vi "parse -- split by line.vi"() -> ()   [LabVIEW 2010]
panel:
  in  "regexp":string="(\\s*[\\d\\.\\+\\-]+)+\\s*\\r?"
  in  "string array":string[](array[string])
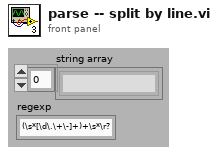
[diagram p1: front panel]
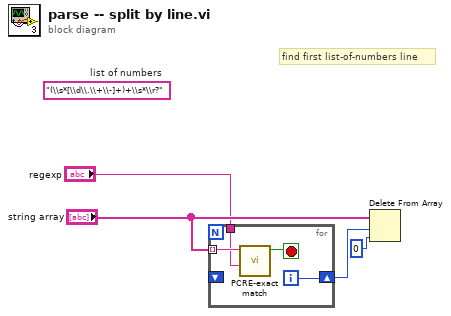
[diagram p0: block diagram]
diagram:
  (unwired) "(\\s*[\\d\\.\\+\\-]+)+\\s*\\r?"  # list of numbers
  # "find first list-of-numbers line"
  n1 = for {
    tunnel: "string array" -> [w8] mode=indexing
    shift-right: [w6] -> w4
    shift-left: _ -> [_]
    tunnel: "regexp" -> [w5]
    i -> [w6]
    stop <- w7 stop-if-true
    n2 = call "PCRE-exact match.vi"("regular expression"=w5, "input string"=w8) -> ("exact match"=w7:bool)  [unwired: 8 in, 1 out]
  }
  n3 = Delete From Array(array="string array", length=w4, index=0 ("index (row)")) -> ()  [unwired: 2 out]
